vi "Configure Hardware.vi"(8 "error in (no error)":errorcluster, 11 "Hardware Resources in":T1={"AIDAQ"="", "Signal Type"=enum."Sine Wave", "DODAQ"=""}) -> (0 "error out":errorcluster, 3 "Hardware Resources out":T1={"AIDAQ"="", "Signal Type"=enum."Sine Wave", "DODAQ"=""})   [LabVIEW 2023, in "Acquisition.lvlib"]
doc: "Configure the hardware."
uses:
  Acquisition.lvlib
  Hardware Configuration.ctl
  Signal Type.ctl
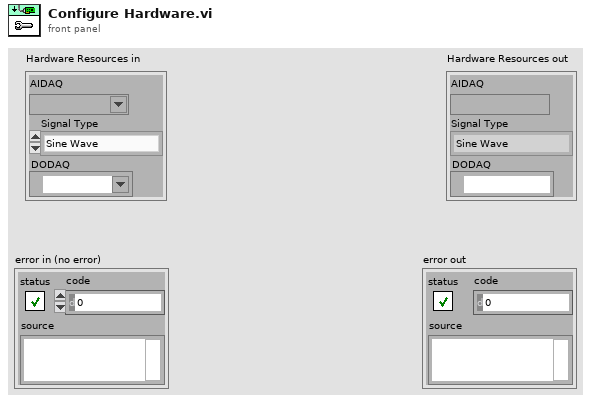
[diagram p1: front panel]
types:
  T1 = typedef "Acquisition.lvlib/Hardware Configuration.ctl" = cluster{"AIDAQ":refnum<k21>, "Signal Type":T2, "DODAQ":refnum<k21>}
  T2 = typedef "Acquisition.lvlib/Signal Type.ctl" = enum16{"cDAQ RTD", "myDAQ Temp", "Sine Wave", "Square with Noise"}
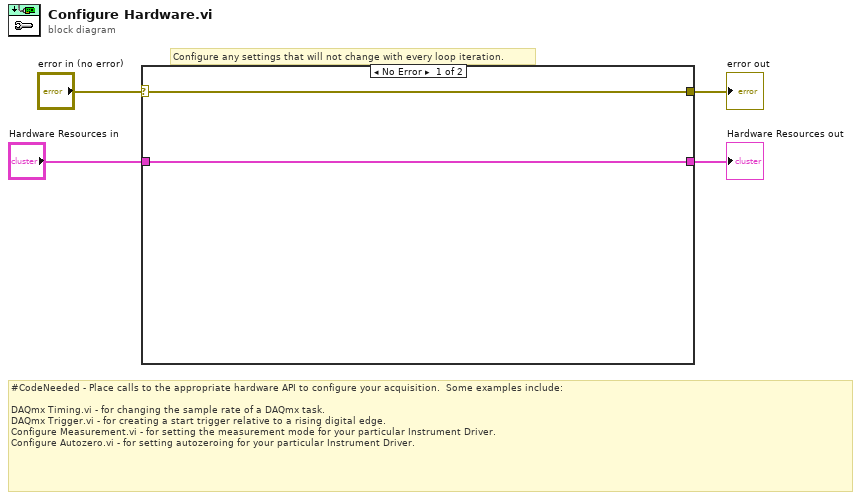
[diagram p0: block diagram]
diagram:
  # "Configure any settings that will not change with every loop iteration."
  # "#CodeNeeded - Place calls to the appropriate hardware API to configure your acquisition.  Some examples include:\n\nDAQmx Timing.vi - for changing the sample rate of a DAQmx task.\nDAQmx Trigger.vi - for creating a start trigger relative to a rising digital edge.\nConfigure Measurement.vi - for setting the measurement mode for your particular Instrument Driver.\nConfigure Autozero.vi - for setting autozeroing for your particular Instrument Driver."
  n1 = case shown="No Error" "error in (no error)" {
    selector: "error in (no error)" -> [w6 w7]
    tunnel: [w6 w7] -> w3
    tunnel: "Hardware Resources in" -> [w5 w8]
    tunnel: [w5 w8] -> w1
    frame No Error {
    }
    frame Error {
    }
  }
  "Hardware Resources out" <- w1
  "error out" <- w3
